vi "New Image.vi"(4 "ImageTimestamp":timestamp, 6 "Camera":string, 8 "error in (no error)":errorcluster, 9 "Buffer Number":u32, 10 "Image":T1, 11 "HIJ Vision Display In":refnum<class "HIJ Vision Display.lvclass">) -> (0 "error out":errorcluster, 3 "HIJ Vision Display Out":refnum<class "HIJ Vision Display.lvclass">)   [LabVIEW 2020, in "HIJ Vision Display.lvlib" / "HIJ Vision Display.lvclass"]
uses:
  HIJ Vision Display.lvclass
  <vilib>/vision/Image Controls.llb/IMAQ Image.ctl
  HIJ Vision Display.lvclass/HIJ Vision Display.ctl
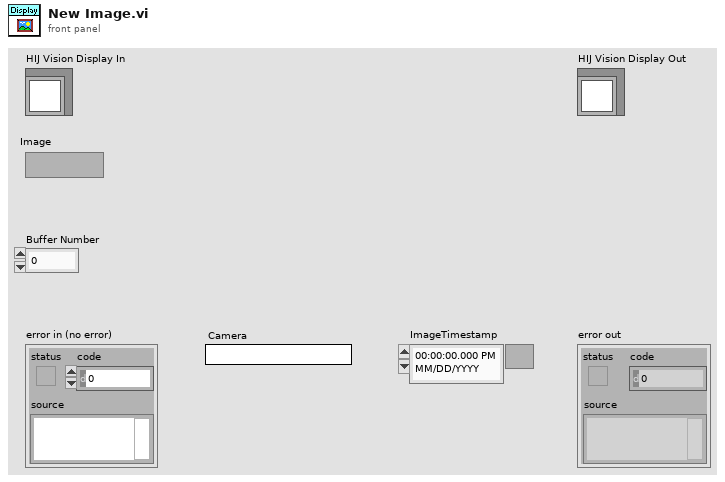
[diagram p1: front panel]
types:
  T1 = typedef "IMAQ Image.ctl" = refnum<image>
  T2 = typedef "Image Type" = u32
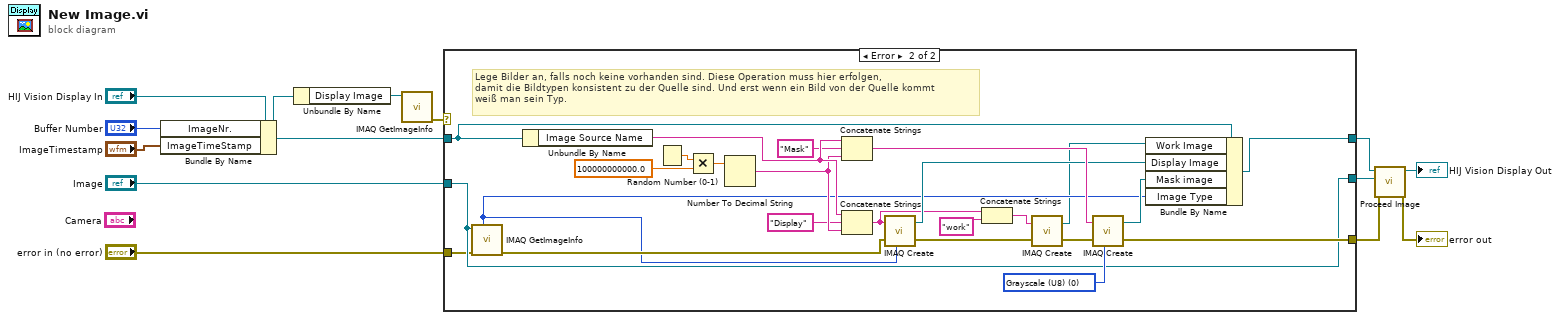
[diagram p0: block diagram]
diagram:
  n1 = Bundle By Name(cluster="HIJ Vision Display In", "ImageNr."="Buffer Number", "ImageTimeStamp"="ImageTimestamp") -> (w6:refnum<class "HIJ Vision Display.lvclass">)
  n2 = Unbundle By Name(w6) -> ("Display Image"=w9:T1)
  n3 = call "IMAQ GetImageInfo"("Image"=w9) -> ("error out"=w8:errorcluster)  [unwired: 3 in, 7 out]
  n4 = case shown="Error" w8 {
    tunnel: [w16 w26] -> w7
    tunnel: w6 -> [w16 w27]
    tunnel: "Image" -> [w15 w25]
    tunnel: [w15 w25] -> w5
    tunnel: "error in (no error)" -> [w14 w24]
    tunnel: [w14 w28] -> w3
    frame No Error {
    }
    frame Error {
      w37 = T2 0 items=["Grayscale (U8)", "Grayscale (I16)", "Grayscale (SGL)", "Complex (CSG)", "RGB (U32)", "HSL (U32)", "RGB (U64)", "Grayscale (U16)"] ("Image Type")
      # "Lege Bilder an, falls noch keine vorhanden sind. Diese Operation muss hier erfolgen,\ndamit die Bildtypen konsistent zu der Quelle sind. Und erst wenn ein Bild von der Quelle kommt\nweiß man sein Typ."
      n5 = call "IMAQ GetImageInfo"("error in (no error)"=w24, "Image"=w25) -> ("error out"=w23:errorcluster, "Image Type"=w22:T2)  [unwired: 2 in, 6 out]
      n6 = Unbundle By Name(w27) -> ("Image Source Name"=w36:string)
      n7 = Random Number (0-1)() -> (number: 0 to 1=w31:dbl)
      n8 = Multiply(x=w31, y=100000000000.0) -> (x*y=w33:dbl)
      n9 = Number To Decimal String(number=w33) -> (decimal integer string=w35:string)  [unwired: 1 in]
      n10 = Concatenate Strings(w36, "Mask" ("string"), w35) -> (w40:string)
      n11 = Concatenate Strings(w36, "Display" ("string"), w35) -> (w17:string)
      n12 = call "IMAQ Create"("Image Name"=w17, "Image Type"=w22, "error in (no error)"=w23) -> ("New Image"=w39:T1, "error out"=w29:errorcluster)  [unwired: 2 in]
      n13 = Concatenate Strings(w17, "work" ("string")) -> (w20:string)
      n14 = call "IMAQ Create"("Image Name"=w20, "error in (no error)"=w29) -> ("New Image"=w18:T1, "error out"=w21:errorcluster)  [unwired: 3 in]
      n15 = call "IMAQ Create"("Image Name"=w40, "Image Type"=w37, "error in (no error)"=w21) -> ("New Image"=w38:T1, "error out"=w28:errorcluster)  [unwired: 2 in]
      n16 = Bundle By Name(cluster=w27, "Work Image"=w18, "Display Image"=w39, "Mask image"=w38, "Image Type"=w22) -> (w26:refnum<class "HIJ Vision Display.lvclass">)
    }
  }
  n17 = call "Proceed Image.vi"("error in (no error)"=w3, "Image"=w5, "IMAQ Display in"=w7) -> ("error out"=→"error out":errorcluster, "HIJ Vision Display out"=→"HIJ Vision Display Out":refnum<class "HIJ Vision Display.lvclass">)  [unwired: 7 in]
